vi "SVT UFF58 Read Record 6.vi"(0 "function refnum":refnum<k20>, 11 "error in (no error)":errorcluster) -> (4 "dup function refnum":refnum<k20>, 6 "DOF identification":T1 {"reference direction" items=["-Z Rotation"=-6, "-Y Rotation"=-5, "-X Rotation"=-4, "-Z Translation"=-3, "-Y Translation"=-2, "-X Translation"=-1, "Scalar"=0, "+X Translation"=1, "+Y Translation"=2, "+Z Translation"=3, "+X Rotation"=4, "+Y Rotation"=5, "+Z Rotation"=6]; "response direction" items=["-Z Rotation"=-6, "-Y Rotation"=-5, "-X Rotation"=-4, "-Z Translation"=-3, "-Y Translation"=-2, "-X Translation"=-1, "Scalar"=0, "+X Translation"=1, "+Y Translation"=2, "+Z Translation"=3, "+X Rotation"=4, "+Y Rotation"=5, "+Z Rotation"=6]}, 15 "error out":errorcluster)   [LabVIEW 2017, in "SoundVib_UFF58.lvlib"]
doc: "Reads the values of all the fields in record 6 of a UFF58 (universal file format) file. Record 6 contains the degree of freedom identification."
uses:
  <vilib>/addons/Sound and Vibration/svt_UFF58/SoundVib_UFF58.lvlib
  <vilib>/addons/Sound and Vibration/svt_UFF58/subVIs/sv_UFF58 DOF.ctl
  <vilib>/addons/Sound and Vibration/svt_UFF58/subVIs/sv_FunctionType.ctl
  <vilib>/addons/Sound and Vibration/svt_UFF58/subVIs/sv_UFF58 Response Direction.ctl
  <vilib>/Platform/storage/Storage.llb/Get Property (String).vi
  <vilib>/Platform/storage/Storage.llb/Get Property (I32).vi
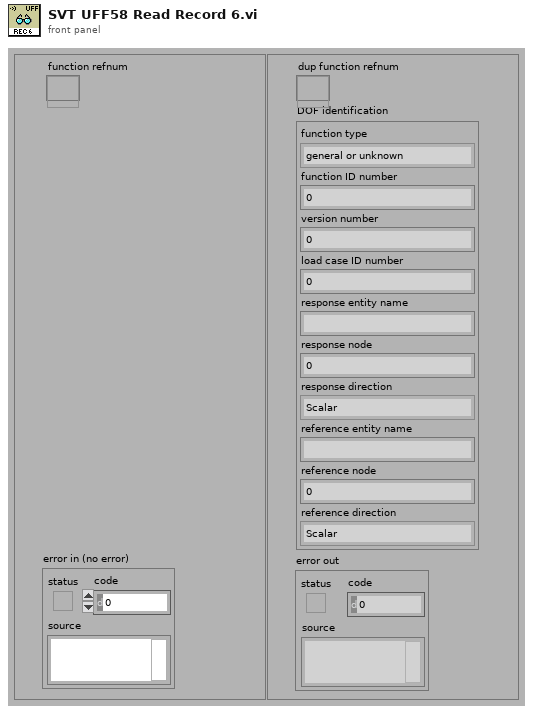
[diagram p1: front panel]
types:
  T1 = typedef "SoundVib_UFF58.lvlib/sv_UFF58 DOF.ctl" = cluster{"function type":T2, "function ID number":i32, "version number":i32, "load case ID number":i32, "response entity name":string, "response node":i32, "response direction":T3, "reference entity name":string, "reference node":i32, "reference direction":T3}
  T2 = typedef "SoundVib_UFF58.lvlib/sv_FunctionType.ctl" = enum16{"general or unknown", "time response", "auto spectrum", "cross spectrum", "frequency response function", "transmissibility", "coherence", "auto correlation", "cross correlation", "power spectral density (PSD)", "energy spectral density (ESD)", "probability density function", "spectrum", "cumulative frequency distribution", "peaks valley", "stress/cycles", "strain/cycles", "orbit", "mode indicator function", "force pattern", "partial power", "partial coherence", "eigenvalue", "eigenvector", "shock response spectrum", "finite impulse response filter", "multiple coherence", "order function", "phase compensation"}
  T3 = typedef "SoundVib_UFF58.lvlib/sv_UFF58 Response Direction.ctl" = i32
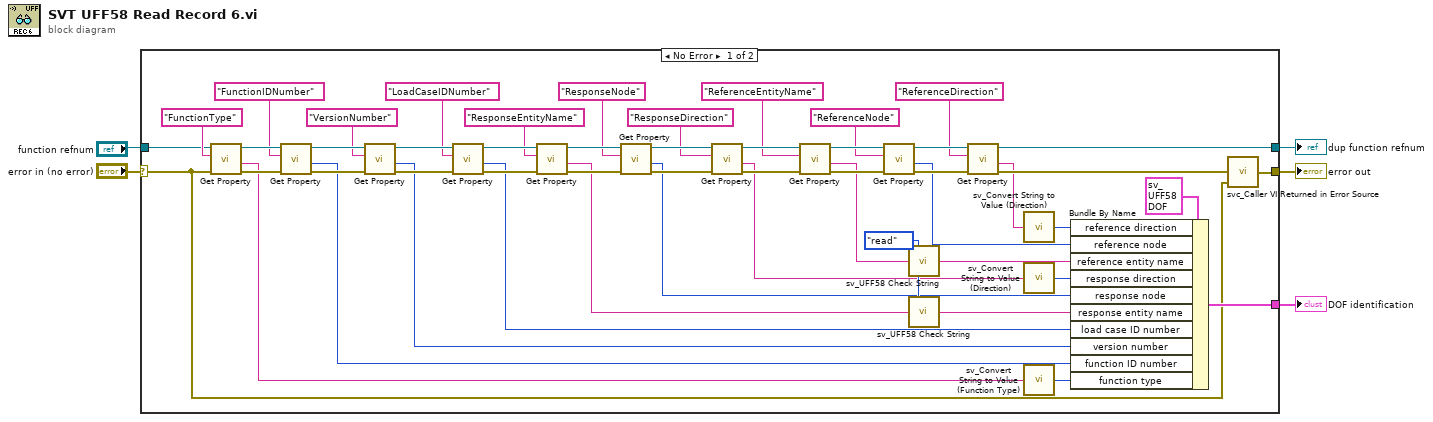
[diagram p0: block diagram]
diagram:
  n1 = case shown="No Error" "error in (no error)" {
    selector: "error in (no error)" -> [w18 w57]
    tunnel: "function refnum" -> [w20 w58]
    tunnel: [w26 w57] -> w5
    tunnel: [w29 w58] -> w3
    tunnel: [w28 _] -> w1
    frame No Error {
      w22 = enum16{"read", "write"}."read" ("operation")
      n2 = call-poly <vilib>:"Get Property.vi"("error in (no error)"=w18, "Property name"="FunctionType", "storage refnum"=w20) -> ("error out"=w55:errorcluster, "Value"=w16:string, "storage refnum out"=w56:refnum<k20>)  [unwired: 6 in]
      n3 = call-poly <vilib>:"Get Property.vi"("error in (no error)"=w55, "Property name"="FunctionIDNumber", "storage refnum"=w56) -> ("error out"=w53:errorcluster, "Value"=w11:i32, "storage refnum out"=w54:refnum<k20>)  [unwired: 6 in]
      n4 = call-poly <vilib>:"Get Property.vi"("error in (no error)"=w53, "Property name"="VersionNumber", "storage refnum"=w54) -> ("error out"=w49:errorcluster, "Value"=w9:i32, "storage refnum out"=w50:refnum<k20>)  [unwired: 6 in]
      n5 = call-poly <vilib>:"Get Property.vi"("error in (no error)"=w49, "Property name"="LoadCaseIDNumber", "storage refnum"=w50) -> ("error out"=w48:errorcluster, "Value"=w7:i32, "storage refnum out"=w47:refnum<k20>)  [unwired: 6 in]
      n6 = call-poly <vilib>:"Get Property.vi"("error in (no error)"=w48, "Property name"="ResponseEntityName", "storage refnum"=w47) -> ("error out"=w46:errorcluster, "Value"=w25:string, "storage refnum out"=w45:refnum<k20>)  [unwired: 6 in]
      n7 = call-poly <vilib>:"Get Property.vi"("error in (no error)"=w46, "Property name"="ResponseNode", "storage refnum"=w45) -> ("error out"=w37:errorcluster, "Value"=w6:i32, "storage refnum out"=w38:refnum<k20>)  [unwired: 6 in]
      n8 = call-poly <vilib>:"Get Property.vi"("error in (no error)"=w37, "Property name"="ResponseDirection", "storage refnum"=w38) -> ("error out"=w40:errorcluster, "Value"=w19:string, "storage refnum out"=w39:refnum<k20>)  [unwired: 6 in]
      n9 = call-poly <vilib>:"Get Property.vi"("error in (no error)"=w40, "Property name"="ReferenceEntityName", "storage refnum"=w39) -> ("error out"=w41:errorcluster, "Value"=w23:string, "storage refnum out"=w42:refnum<k20>)  [unwired: 6 in]
      n10 = call-poly <vilib>:"Get Property.vi"("error in (no error)"=w41, "Property name"="ReferenceNode", "storage refnum"=w42) -> ("error out"=w43:errorcluster, "Value"=w12:i32, "storage refnum out"=w44:refnum<k20>)  [unwired: 6 in]
      n11 = call <vilib>:"sv_UFF58 Check String.vi"("operation"=w22, "field value"=w23) -> ("output string"=w10:string)  [unwired: 12 in, 1 out]
      n12 = call <vilib>:"sv_UFF58 Check String.vi"("operation"=w22, "field value"=w25) -> ("output string"=w24:string)  [unwired: 12 in, 1 out]
      n13 = call-poly <vilib>:"Get Property.vi"("error in (no error)"=w43, "Property name"="ReferenceDirection", "storage refnum"=w44) -> ("error out"=w27:errorcluster, "Value"=w17:string, "storage refnum out"=w29:refnum<k20>)  [unwired: 6 in]
      n14 = call <vilib>:"sv_Convert String to Value (Direction).vi"("direction string"=w17) -> ("direction value"=w14:T3)  [unwired: 14 in]
      n15 = call <vilib>:"sv_Convert String to Value (Direction).vi"("direction string"=w19) -> ("direction value"=w8:T3)  [unwired: 14 in]
      n16 = call <vilib>:"sv_Convert String to Value (Function Type).vi"("function type string"=w16) -> ("function type value"=w13:T2)  [unwired: 14 in]
      n17 = Bundle By Name(cluster=T1 {"function type"=enum."general or unknown", "function ID number"=0, "version number"=0, "load case ID number"=0, "response entity name"="", "response node"=0, "response direction"=0, "reference entity name"="", "reference node"=0, "reference direction"=0} ("DOF identification"), "reference direction"=w14, "reference node"=w12, "reference entity name"=w10, "response direction"=w8, "response node"=w6, "response entity name"=w24, "load case ID number"=w7, "version number"=w9, "function ID number"=w11, "function type"=w13) -> (w28:T1)
      n18 = call <vilib>:"svc_Caller VI Returned in Error Source.vi"("warning input to caller"=w18, "error in (no error)"=w27) -> ("error out"=w26:errorcluster)  [unwired: 3 in]
    }
    frame Error {
    }
  }
  "error out" <- w5
  "DOF identification" <- w1
  "dup function refnum" <- w3
